vi "pop next connection.vi"(8 "error in":errorcluster, 11 "connection creator in":refnum<class "connection creator.lvclass">) -> (0 "error out":errorcluster, 3 "connection out":refnum<class "connection.lvclass">)   [LabVIEW 2016, in "connection creator.lvclass"]
uses:
  connection creator.lvclass
  connection/connection.lvclass
  connection creator.lvclass/connection creator.ctl
  dllwrapper/library path.vi
  dllwrapper/dispose socket.vi
  dllwrapper/async tls dl.lvlib
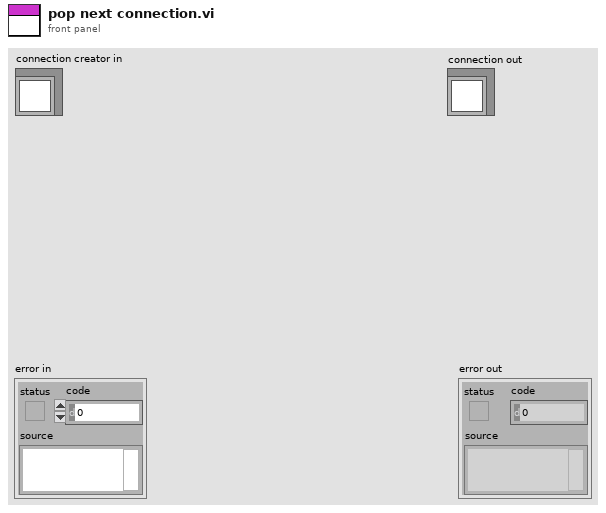
[diagram p1: front panel]
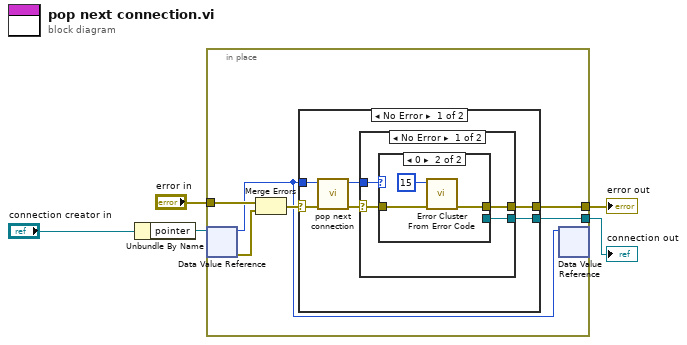
[diagram p0: block diagram]
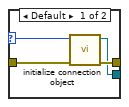
[diagram p2: hidden frame]
diagram:
  n1 = Unbundle By Name("connection creator in") -> ("pointer"=w3:refnum<data-value>)
  n2 = in-place {
    in-place-border: "error in" -> [w10]
    in-place-border: [w8] -> w2
    in-place-border: [w6] -> w1
    n3 = in-place-dvr #1(w3) -> (w7:u64, w11:errorcluster)
    n4 = Merge Errors(w10, w11) -> (w9:errorcluster)
    n5 = case shown="No Error" w9 {
      selector: w9 -> [w17 w30]
      tunnel: [w14 w30] -> w8
      tunnel: w7 -> [w16 _]
      tunnel: [w12 _] -> w6
      frame No Error {
        n6 = call "pop next connection.vi"("error in"=w17, "conn creator"=w16) -> ("error out"=w15:errorcluster, "connection handle"=w13:u64)  [unwired: 8 in]
        n7 = case shown="No Error" w15 {
          selector: w15 -> [w20 w29]
          tunnel: [w19 w29] -> w14
          tunnel: w13 -> [w21 _]
          tunnel: [w18 _] -> w12
          frame No Error {
            n8 = case shown="0" w21 {
              selector: w21 -> [w25 _]
              tunnel: w20 -> [w24 w27]
              tunnel: [w23 w26] -> w19
              tunnel: [w22 _] -> w18
              frame Default {
                n9 = call "initialize connection object.vi"("error in"=w24, "connection"=w25) -> ("error out"=w23:errorcluster, "connection out"=w22:refnum<class "connection.lvclass">)  [unwired: 8 in]
              }
              frame 0 {
                n10 = call <vilib>:"Error Cluster From Error Code.vi"("error in (no error)"=w27, "error code (0)"=15) -> ("error out"=w26:errorcluster)  [unwired: 7 in]
              }
            }
          }
          frame Error {
          }
        }
      }
      frame Error {
      }
    }
    n11 = in-place-dvr #1(w7) -> ()  [unwired: 2 out]
  }
  "error out" <- w2
  "connection out" <- w1
